vi "DataSimulation.vi"(3 "PWM Input [0-2200]":dbl) -> (0 "Amp Draw from Ammeter [Volts]":dbl, 1 "Thrust from Force Gauge":dbl)   [LabVIEW 2015]
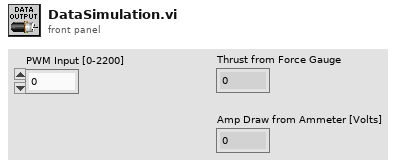
[diagram p1: front panel]
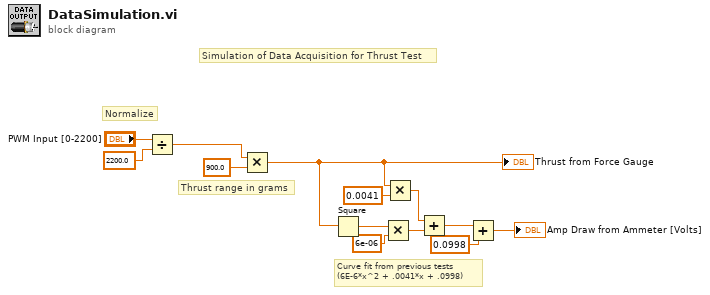
[diagram p0: block diagram]
diagram:
  # "Simulation of Data Acquisition for Thrust Test"
  # "Curve fit from previous tests\n(6E-6*x^2 + .0041*x + .0998)"
  # "Thrust range in grams"
  # "Normalize"
  n1 = Divide(x="PWM Input [0-2200]", y=2200.0) -> (x/y=w10:dbl)
  n2 = Multiply(x=w10, y=900.0) -> (x*y=w2:dbl)
  "Thrust from Force Gauge" <- w2
  n3 = Square(x=w2) -> (x^2=w8:dbl)
  n4 = Multiply(x=w8, y=6e-06) -> (x*y=w7:dbl)
  n5 = Multiply(x=w2, y=0.0041) -> (x*y=w3:dbl)
  n6 = Add(x=w3, y=w7) -> (x+y=w5:dbl)
  n7 = Add(x=w5, y=0.0998) -> (x+y=→"Amp Draw from Ammeter [Volts]":dbl)
